vi "Rinse Channel.vi"(8 "error in (no error)":errorcluster, 11 "Rinse volume":dbl=250.0 format="%#_g uL") -> (0 "error out":errorcluster)   [LabVIEW 2018, in "cetoni.lvlib" / "cetoni.lvclass"]
uses:
  cetoni.lvclass
  Resources/GLOBAL/GLOBAL Time-critical.vi
  <userlib>/QmixLib/QmixLib.lvlib
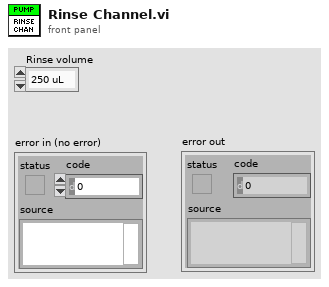
[diagram p1: front panel]
types:
  T1 = enum16{"LOW_PRESSURE_VALVE", "BALL_VALVE", "QMIX_VALVE"}
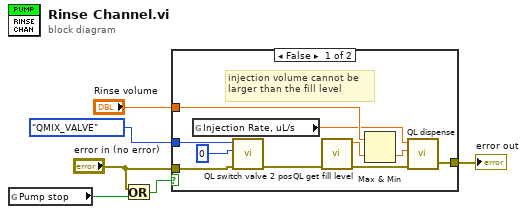
[diagram p0: block diagram]
diagram:
  n1 = global read "GLOBAL Time-critical.vi" "Pump stop"() -> (w3:bool)
  n2 = Or(x="error in (no error)", y=w3) -> (x .or. y?=w2:bool)
  n3 = case shown="False" w2 {
    tunnel: [w16 w17] -> w6
    tunnel: "Rinse volume" -> [w12 _]
    tunnel: T1."QMIX_VALVE" ("valve") -> [w9 _]
    tunnel: "error in (no error)" -> [w7 w17]
    frame False {
      # "injection volume cannot be\nlarger than the fill level"
      n4 = global read "GLOBAL Time-critical.vi" "Injection Rate, uL/s"() -> (w11:dbl)
      n5 = call <userlib>:"QL switch valve 2 pos.vi"("error in (no error)"=w7, "pos"=0, "valve"=w9) -> ("error out"=w10:errorcluster)  [unwired: 8 in]
      n6 = call <userlib>:"QL get fill level.vi"("error in (no error)"=w10) -> ("error out"=w13:errorcluster, "Fill level, uL"=w15:dbl)  [unwired: 9 in]
      n7 = Max & Min(x=w12, y=w15) -> (min(x,y)=w14:dbl)  [unwired: 1 out]
      n8 = call <userlib>:"QL dispense.vi"("error in (no error)"=w13, "volume_uL"=w14, "flow_rate_uL_s"=w11) -> ("error out"=w16:errorcluster)  [unwired: 4 in]
    }
    frame True {
    }
  }
  "error out" <- w6
